vi "Begin.vi"(8 "error in (no error)":errorcluster, 10 "Configuration in":variant, 11 "Power Cell Handler in":refnum<class "Power Cell Handler.lvclass">) -> (0 "error out":errorcluster, 3 "Power Cell Handler out":refnum<class "Power Cell Handler.lvclass">)   [LabVIEW 2019, in "Power Cell Handler.lvlib" / "Power Cell Handler.lvclass"]
uses:
  Power Cell Handler.lvclass
  <vilib>/Rock Robotics/WPI/ThirdParty/Phoenix-LabVIEW/Motor Controller/Controls/CTRE_Phoenix_MotorControl_SupplyCurrentLimitConfiguration.ctl
  Power Cell Handler.lvclass/Power Cell Handler.ctl
  <vilib>/Rock Robotics/WPI/ThirdParty/Phoenix-LabVIEW/Motor Controller/Controls/CTRE_Phoenix_MotorControl_FeedbackDevice_TalonFX.ctl
  <vilib>/Rock Robotics/WPI/ThirdParty/Phoenix-LabVIEW/Motor Controller/Controls/CTRE_Phoenix_MotorControl_TalonFXInvertType.ctl
  <vilib>/Rock Robotics/WPI/ThirdParty/Phoenix-LabVIEW/Motor Controller/Controls/CTRE_Phoenix_MotorControl_FeedbackDevice.ctl
  7b361c19-ac6e-4022-bfe1-45901947c1fc.vi
  19b491db-85f4-4e91-bd7a-c7c0939619b7.vi
  10e73dc3-d3e9-4580-8caf-7344cce1af74.vi
  ea745d27-1b7a-4aa6-8db5-1ac96fa4d0e2.vi
  80b243bf-0e5b-4295-a3d8-317614f9daec.vi
  7ce307d2-5cf6-42cf-8e64-50757e446175.vi
  680ce7d0-c1b2-4c80-9ba9-9f229533ea2f.vi
  848b9887-b104-4cac-9511-37ed5d87697b.vi
  <vilib>/Utility/error.llb/Trim Whitespace.vi
  <vilib>/Utility/error.llb/Error Cluster From Error Code.vi
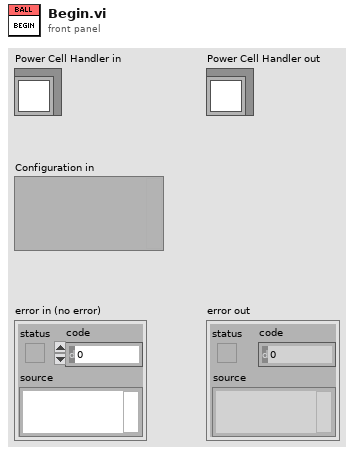
[diagram p1: front panel]
types:
  T1 = typedef "CTRE_Phoenix_MotorControl_SupplyCurrentLimitConfiguration.ctl" = cluster{"Enable?":bool, "Current Limit":dbl, "Threshold Current":dbl, "Threshold Time":dbl}
  T2 = typedef "CTRE_Phoenix_MotorControl_TalonFXInvertType.ctl" = enum16{"Counter-Clockwise", "Clockwise"}
  T3 = typedef "CTRE_Phoenix_MotorControl_FeedbackDevice_TalonFX.ctl" = i8
  T4 = typedef "WPI_MotorControlDeviceRef.ctl" = cluster{"DeviceStatus":errorcluster, "Type":T5, "PWM":cluster{"PWM Channel":T6, "DeadBand":T7}, "CAN":cluster{"Device Number":u8, "SetOutput VI Ref":variant, "GetOutput VI Ref":variant, "Enable VI Ref":variant, "Disable VI Ref":variant, "Data":variant}, "Invert":bool, "DIO PWM":cluster{"PWM \"Enable\" Channel":T6, "DIOChannel":T8, "PWM Rate":dbl}}
  T5 = typedef "WPI_MotorControlType.ctl" = enum16{"PWM", "CAN", "DIO PWM"}
  T6 = typedef "FPGA_DIOPWMChannel.ctl" = enum8{"PWM 0", "PWM 1", "PWM 2", "PWM 3", "PWM 4", "PWM 5", "PWM 6", "PWM 7", "PWM 8", "PWM 9", "PWM MXP 0", "PWM MXP 1", "PWM MXP 2", "PWM MXP 3", "PWM MXP 4", "PWM MXP 5", "PWM MXP 6", "PWM MXP 7", "PWM MXP 8", "PWM MXP 9", "Invalid"}
  T7 = typedef "WPI_PWMDeadband.ctl" = cluster{"Name":string, "maxPositivePwm":i32, "minPositivePwm":i32, "centerPwm":i32, "maxNegativePwm":i32, "minNegativePwm":i32, "angularRange":u16}
  T8 = typedef "FPGA_DIOChannel.ctl" = enum8{"DIO 0", "DIO 1", "DIO 2", "DIO 3", "DIO 4", "DIO 5", "DIO 6", "DIO 7", "DIO 8", "DIO 9", "DIO MXP 0", "DIO MXP 1", "DIO MXP 2", "DIO MXP 3", "DIO MXP 4", "DIO MXP 5", "DIO MXP 6", "DIO MXP 7", "DIO MXP 8", "DIO MXP 9", "DIO MXP 10", "DIO MXP 11", "DIO MXP 12", "DIO MXP 13", "DIO MXP 14", "DIO MXP 15", "SPI Port CS1", "SPI Port CS2", "SPI Port CS3", "SPI Port MISO", "SPI Port MOSI", "Invalid"}
  T9 = typedef "CTRE_Phoenix_MotorControl_FeedbackDevice.ctl" = i8
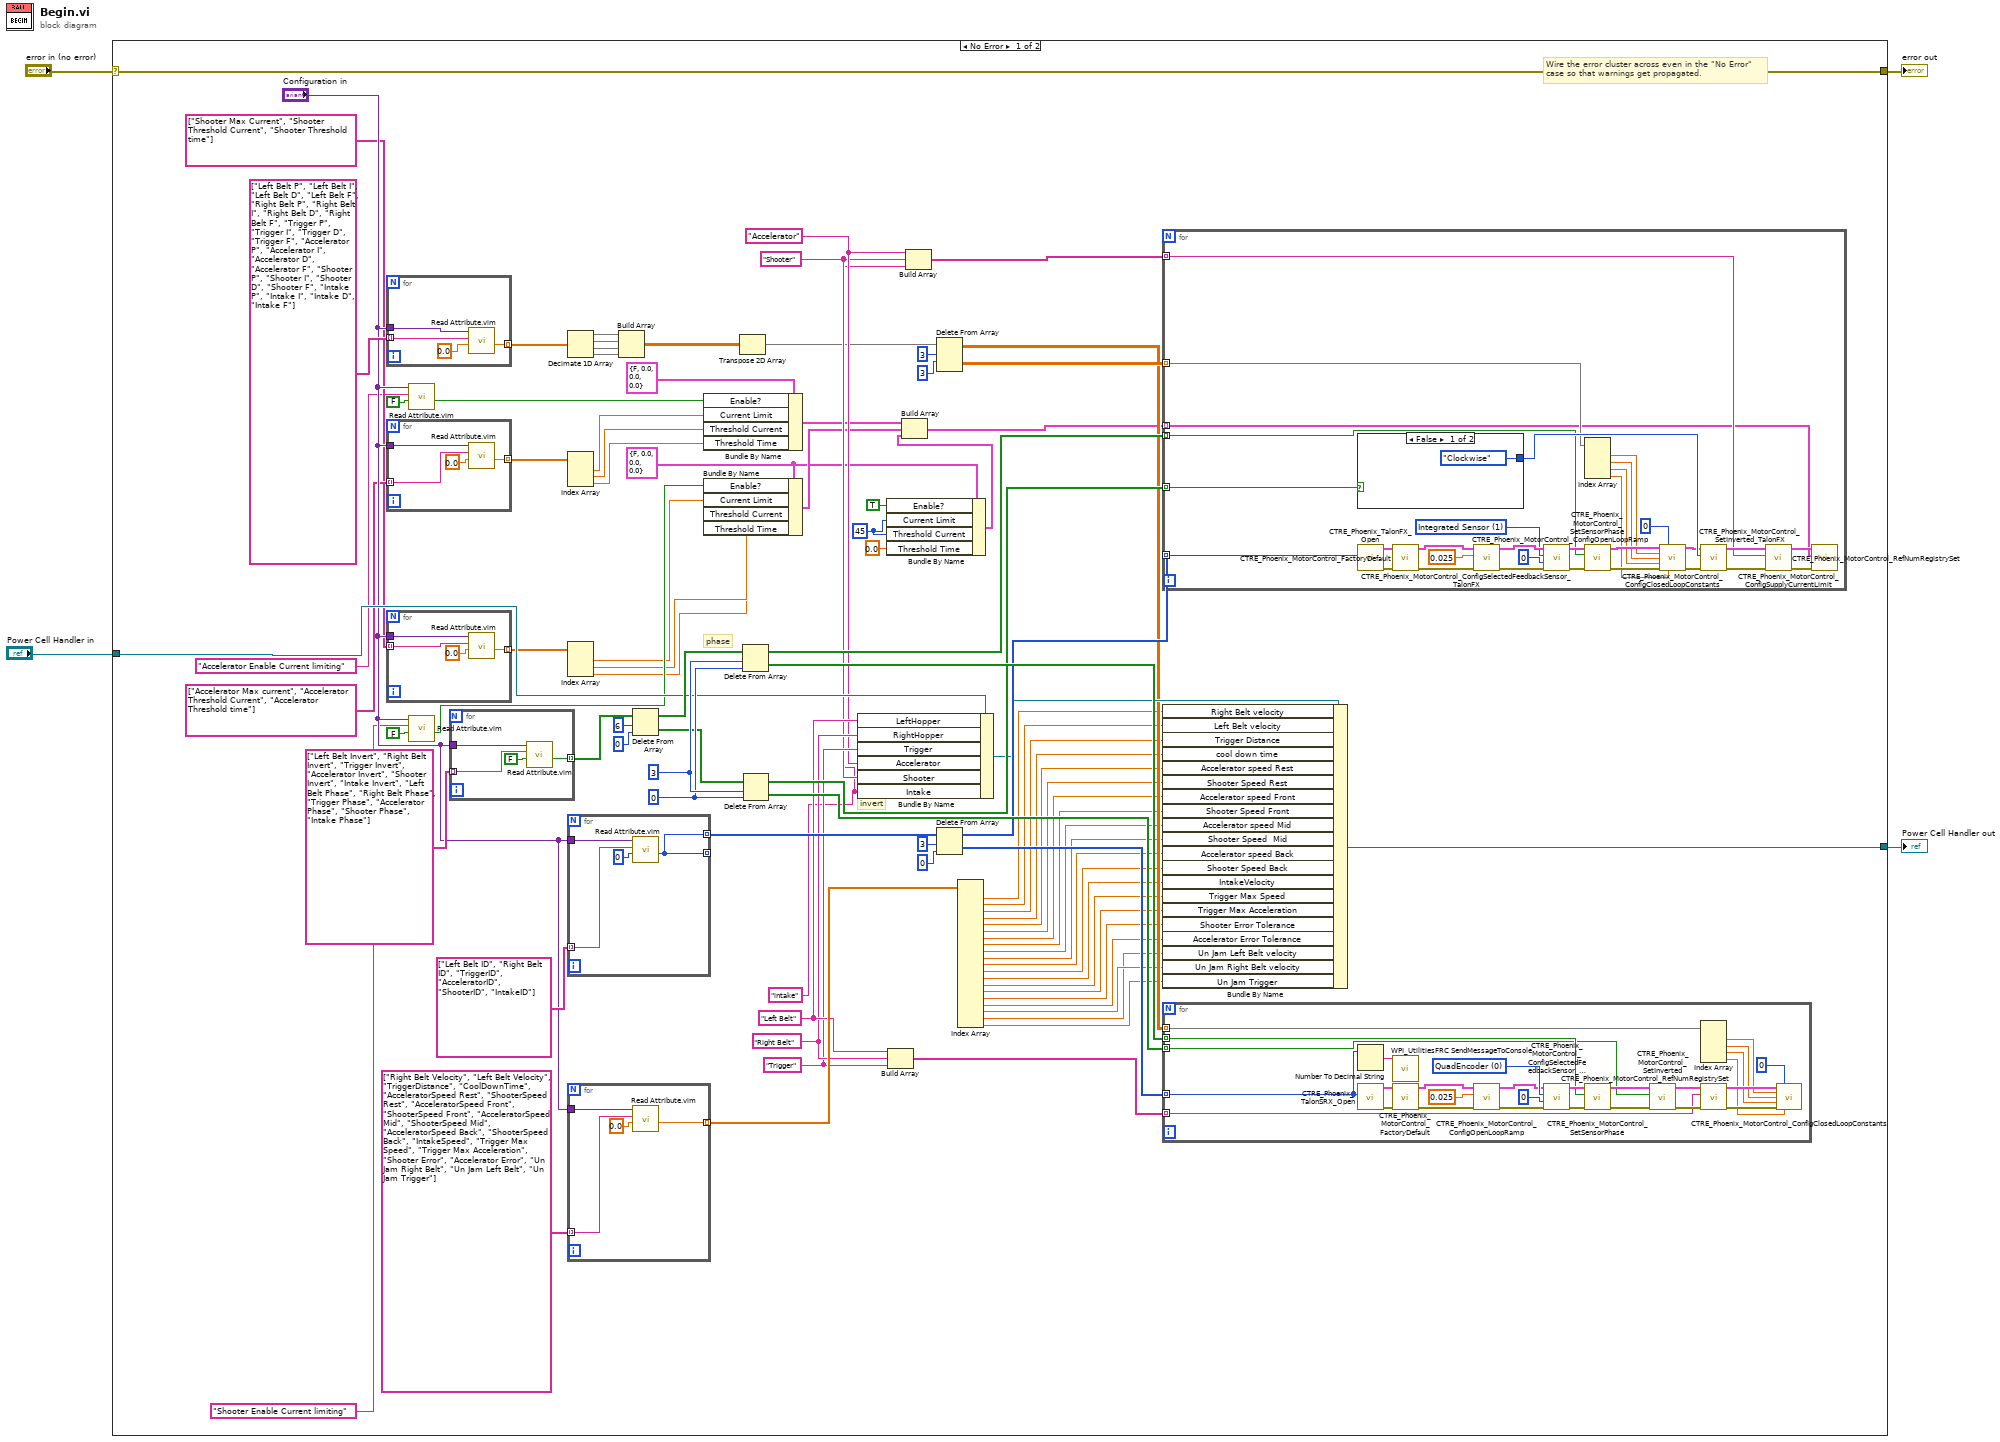
[diagram p0: block diagram]
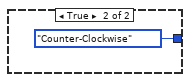
[diagram p2: hidden frame]
diagram:
  n1 = case shown="No Error" "error in (no error)" {
    selector: "error in (no error)" -> [w94 w181]
    tunnel: [w94 w181] -> w3
    tunnel: [w63 w180] -> w1
    tunnel: "Power Cell Handler in" -> [w72 w180]
    frame No Error {
      w8 = 45
      w10 = T1 {"Enable?"=FALSE, "Current Limit"=0.0, "Threshold Current"=0.0, "Threshold Time"=0.0} ("Supply Current Limit Configuration 2")
      w5 = "intake"
      w65 = "Shooter"
      w66 = "Accelerator"
      w68 = "Trigger"
      w69 = "Right Belt"
      w70 = "Left Belt"
      w87 = 3 ("length")
      w86 = 0 ("index")
      # "phase"
      # "invert"
      # "Wire the error cluster across even in the \"No Error\"\ncase so that warnings get propagated."
      n2 = for {
        tunnel: "Configuration in" -> [w118]
        tunnel: string[] ["Left Belt P", "Left Belt I", "Left Belt D", "Left Belt F", "Right Belt P", "Right Belt I", "Right Belt D", "Right Belt F", "Trigger P", "Trigger I", "Trigger D", "Trigger F", "Accelerator P", "Accelerator I", "Accelerator D", "Accelerator F", "Shooter P", "Shooter I", "Shooter D", "Shooter F", "Intake P", "Intake I", "Intake D", "Intake F"] -> [w117] mode=indexing
        tunnel: [w116] -> w62 mode=indexing
        n3 = call "Read Attribute.vim"("default value (data type)"=0.0, "name"=w117, "variant in"=w118) -> ("value"=w116:dbl)  [unwired: 5 in, 3 out]
      }
      n4 = for {
        tunnel: "Configuration in" -> [w102]
        tunnel: [w101] -> w37 mode=indexing
        tunnel: string[] ["Accelerator Max current", "Accelerator Threshold Current", "Accelerator Threshold time"] -> [w99] mode=indexing
        n5 = call "Read Attribute.vim"("default value (data type)"=0.0, "name"=w99, "variant in"=w102) -> ("value"=w101:dbl)  [unwired: 5 in, 3 out]
      }
      n6 = for {
        tunnel: "Configuration in" -> [w98]
        tunnel: [w97] -> w36 mode=indexing
        tunnel: string[] ["Shooter Max Current", "Shooter Threshold Current", "Shooter Threshold time"] -> [w95] mode=indexing
        n7 = call "Read Attribute.vim"("default value (data type)"=0.0, "name"=w95, "variant in"=w98) -> ("value"=w97:dbl)  [unwired: 5 in, 3 out]
      }
      n8 = call "Read Attribute.vim"("default value (data type)"=FALSE, "name"="Accelerator Enable Current limiting", "variant in"="Configuration in") -> ("value"=w30:bool)  [unwired: 5 in, 3 out]
      n9 = call "Read Attribute.vim"("default value (data type)"=FALSE, "name"="Shooter Enable Current limiting", "variant in"="Configuration in") -> ("value"=w29:bool)  [unwired: 5 in, 3 out]
      n10 = for {
        tunnel: "Configuration in" -> [w114]
        tunnel: string[] ["Left Belt Invert", "Right Belt Invert", "Trigger Invert", "Accelerator Invert", "Shooter Invert", "Intake Invert", "Left Belt Phase", "Right Belt Phase", "Trigger Phase", "Accelerator Phase", "Shooter Phase", "Intake Phase"] -> [w113] mode=indexing
        tunnel: [w111] -> w91 mode=indexing
        n11 = call "Read Attribute.vim"("default value (data type)"=FALSE, "name"=w113, "variant in"=w114) -> ("value"=w111:bool)  [unwired: 5 in, 3 out]
      }
      n12 = Decimate 1D Array(w62) -> (w61:dbl[], w60:dbl[], w59:dbl[], w46:dbl[])
      n13 = Index Array(array=w37) -> (element #1=w33:dbl, element #2=w32:dbl, element #3=w31:dbl)  [unwired: 3 in]
      n14 = Index Array(array=w36) -> (element #1=w28:dbl, element #2=w27:dbl, element #3=w26:dbl)  [unwired: 3 in]
      n15 = for {
        tunnel: "Configuration in" -> [w110]
        tunnel: string[] ["Left Belt ID", "Right Belt ID", "TriggerID", "AcceleratorID", "ShooterID", "IntakeID"] -> [w109] mode=indexing
        tunnel: [w108] -> _ mode=indexing
        tunnel: [w108] -> w79 mode=indexing
        n16 = call "Read Attribute.vim"("default value (data type)"=0, "name"=w109, "variant in"=w110) -> ("value"=w108:i32)  [unwired: 5 in, 3 out]
      }
      n17 = for {
        tunnel: "Configuration in" -> [w106]
        tunnel: string[] ["Right Belt Velocity", "Left Belt Velocity", "TriggerDistance", "CoolDownTime", "AcceleratorSpeed Rest", "ShooterSpeed Rest", "AcceleratorSpeed Front", "ShooterSpeed Front", "AcceleratorSpeed Mid", "ShooterSpeed Mid", "AcceleratorSpeed Back", "ShooterSpeed Back", "IntakeSpeed", "Trigger Max Speed", "Trigger Max Acceleration", "Shooter Error", "Accelerator Error", "Un Jam Right Belt", "Un Jam Left Belt", "Un Jam Trigger"] -> [w105] mode=indexing
        tunnel: [w104] -> w73 mode=indexing
        n18 = call "Read Attribute.vim"("default value (data type)"=0.0, "name"=w105, "variant in"=w106) -> ("value"=w104:dbl)  [unwired: 5 in, 3 out]
      }
      n19 = Build Array(w61, w60, w59, w46) -> (w58:dbl[][])
      n20 = Delete From Array(array=w91, length=6, index=0) -> (deleted portion=w85:bool[], array with subset deleted=w88:bool[])
      n21 = Bundle By Name(cluster=T1 {"Enable?"=FALSE, "Current Limit"=0.0, "Threshold Current"=0.0, "Threshold Time"=0.0} ("Supply Current Limit Configuration"), "Enable?"=w30, "Current Limit"=w33, "Threshold Current"=w32, "Threshold Time"=w31) -> (w35:T1)
      n22 = Bundle By Name(cluster=w10, "Enable?"=w29, "Current Limit"=w28, "Threshold Current"=w27, "Threshold Time"=w26) -> (w34:T1)
      n23 = Transpose 2D Array(2D array=w58) -> (transposed array=w53:dbl[][])
      n24 = Delete From Array(array=w88, length=w87, index=w86) -> (deleted portion=w83:bool[], array with subset deleted=w81:bool[])
      n25 = Delete From Array(array=w85, length=w87, index=w86) -> (deleted portion=w84:bool[], array with subset deleted=w82:bool[])
      n26 = Bundle By Name(cluster=w72, "LeftHopper"=w70, "RightHopper"=w69, "Trigger"=w68, "Accelerator"=w66, "Shooter"=w65, "Intake"=w5) -> (w71:refnum<class "Power Cell Handler.lvclass">)
      n27 = Bundle By Name(cluster=w10, "Enable?"=TRUE, "Current Limit"=w8, "Threshold Current"=w8, "Threshold Time"=0.0) -> (w6:T1)
      n28 = Build Array(w70, w69, w68) -> (w67:string[])
      n29 = Build Array(w35, w34, w6) -> (w25:T1[])
      n30 = Build Array(w66, w65, w5) -> (w64:string[])
      n31 = Delete From Array(array=w53, length=3, index (row)=3) -> (deleted portion=w55:dbl[][], array with subset deleted=w54:dbl[][])  [unwired: 1 in]
      n32 = Delete From Array(array=w79, length=3, index=0) -> (deleted portion=w76:i32[], array with subset deleted=w75:i32[])
      n33 = Index Array(array=w73) -> (element #1=w52:dbl, element #2=w51:dbl, element #3=w50:dbl, element #4=w49:dbl, element #5=w48:dbl, element #6=w47:dbl, element #7=w24:dbl, element #8=w23:dbl, element #9=w22:dbl, element #10=w21:dbl, element #11=w20:dbl, element #12=w19:dbl, element #13=w18:dbl, element #14=w17:dbl, element #15=w16:dbl, element #16=w15:dbl, element #17=w14:dbl, element #18=w13:dbl, element #19=w12:dbl, element #20=w11:dbl)  [unwired: 20 in]
      n34 = for {
        tunnel: w55 -> [w127] mode=indexing
        tunnel: w82 -> [w126] mode=indexing
        tunnel: w81 -> [w125] mode=indexing
        tunnel: w75 -> [w124] mode=indexing
        tunnel: w64 -> [w123] mode=indexing
        tunnel: w25 -> [w119] mode=indexing
        w122 = T3 1 items=["Integrated Sensor"=1, "Sensor Sum (S0 + S1)"=9, "Sensor Difference (D0 - D1)"=10, "Remote Source 0"=11, "Remote Source 1"=12, "None"=14, "Software Emulated"=15] ("Talon FX Feedback Device")
        n35 = case shown="False" w126 {
          tunnel: [CTRE_Phoenix_MotorControl_TalonFXInvertType."Clockwise" ("Invert Type") CTRE_Phoenix_MotorControl_TalonFXInvertType."Counter-Clockwise" ("Invert Type")] -> w137
          frame False {
          }
          frame True {
          }
        }
        n36 = call <vilib>:"CTRE_Phoenix_TalonFX_Open.vi"("Device Number"=w124) -> ("error out"=w149:errorcluster, "CAN Talon SRX Ref"=w148:T4)  [unwired: 9 in]
        n37 = call <vilib>:"CTRE_Phoenix_MotorControl_FactoryDefault.vi"("error in"=w149, "PhoenixMotorControlDevRef"=w148) -> ("error out"=w142:errorcluster, "PhoenixMotorControlDevRef"=w143:T4)  [unwired: 8 in]
        n38 = call <vilib>:"CTRE_Phoenix_MotorControl_ConfigOpenLoopRamp.vi"("error in (no error)"=w142, "secondsFromNeutralToFull"=0.025, "PhoenixMotorControlDevRef"=w143) -> ("error out"=w140:errorcluster, "PhoenixMotorControlDevRef"=w141:T4)  [unwired: 7 in]
        n39 = call <vilib>:"CTRE_Phoenix_MotorControl_ConfigSelectedFeedbackSensor_TalonFX.vi"("error in (no error)"=w140, "pidLoopIdx"=0, "Talon FX Feedback Device"=w122, "PhoenixMotorControlDevRef"=w141) -> ("error out"=w145:errorcluster, "PhoenixMotorControlDevRef"=w146:T4)  [unwired: 6 in]
        n40 = Index Array(array=w127) -> (element #1=w131:dbl, element #2=w130:dbl, element #3=w129:dbl, element #4=w128:dbl)  [unwired: 4 in]
        n41 = call <vilib>:"CTRE_Phoenix_MotorControl_SetSensorPhase.vi"("error in (no error)"=w145, "PhaseSensor"=w125, "PhoenixMotorControlDevRef"=w146) -> ("error out"=w135:errorcluster, "PhoenixMotorControlDevRef"=w136:T4)  [unwired: 7 in]
        n42 = call <vilib>:"CTRE_Phoenix_MotorControl_ConfigClosedLoopConstants.vi"("PhoenixMotorControlDevRef"=w136, "slotIdx"=0, "P"=w131, "I"=w130, "D"=w129, "error in (no error)"=w135, "F"=w128) -> ("PhoenixMotorControlDevRef"=w134:T4, "error out"=w133:errorcluster)  [unwired: 7 in]
        n43 = call <vilib>:"CTRE_Phoenix_MotorControl_SetInverted_TalonFX.vi"("error in (no error)"=w133, "Invert Type"=w137, "PhoenixMotorControlDevRef"=w134) -> ("error out"=w139:errorcluster, "PhoenixMotorControlDevRef"=w138:T4)  [unwired: 7 in]
        n44 = call <vilib>:"CTRE_Phoenix_MotorControl_RefNumRegistrySet.vi"("error in (no error)"=w139, "refnum name"=w123, "PhoenixMotorControlDevRef"=w138) -> ("error out"=w120:errorcluster, "PhoenixMotorControlDevRef"=w121:T4)  [unwired: 7 in]
        n45 = call <vilib>:"CTRE_Phoenix_MotorControl_ConfigSupplyCurrentLimit.vi"("error in (no error)"=w120, "Supply Current Limit Configuration"=w119, "PhoenixMotorControlDevRef"=w121) -> ()  [unwired: 7 in, 2 out]
      }
      n46 = Bundle By Name(cluster=w71, "Right Belt velocity"=w52, "Left Belt velocity"=w51, "Trigger Distance"=w50, "cool down time"=w49, "Accelerator speed Rest"=w48, "Shooter Speed Rest"=w47, "Accelerator speed Front"=w24, "Shooter Speed Front"=w23, "Accelerator speed Mid"=w22, "Shooter Speed  Mid"=w21, "Accelerator speed Back"=w20, "Shooter Speed Back"=w19, "IntakeVelocity"=w18, "Trigger Max Speed"=w17, "Trigger Max Acceleration"=w16, "Shooter Error Tolerance"=w15, "Accelerator Error Tolerance"=w14, "Un Jam Left Belt velocity"=w12, "Un Jam Right Belt velocity"=w13, "Un Jam Trigger"=w11) -> (w63:refnum<class "Power Cell Handler.lvclass">)
      n47 = for {
        tunnel: w84 -> [w156] mode=indexing
        tunnel: w83 -> [w157] mode=indexing
        tunnel: w54 -> [w155] mode=indexing
        tunnel: w76 -> [w153] mode=indexing
        tunnel: w67 -> [w154] mode=indexing
        w177 = T9 0 items=["QuadEncoder"=0, "Analog"=2, "Tachometer"=4, "Pulse Width Encoded Position"=8, "Sensor Sum (S0 + S1)"=9, "Sensor Difference (D0 - D1)"=10, "Remote Source 0"=11, "Remote Source 1"=12, "Software Emulated"=15] ("Feedback Device")
        n48 = Number To Decimal String(number=w153) -> (decimal integer string=w152:string)  [unwired: 1 in]
        n49 = call <vilib>:"CTRE_Phoenix_TalonSRX_Open.vi"("Device Number"=w153) -> ("error out"=w176:errorcluster, "CAN Talon SRX Ref"=w175:T4)  [unwired: 9 in]
        n50 = call <vilib>:"WPI_UtilitiesFRC SendMessageToConsole.vi"("Message"=w152) -> ()  [unwired: 14 in, 1 out]
        n51 = call <vilib>:"CTRE_Phoenix_MotorControl_FactoryDefault.vi"("error in"=w176, "PhoenixMotorControlDevRef"=w175) -> ("error out"=w167:errorcluster, "PhoenixMotorControlDevRef"=w168:T4)  [unwired: 8 in]
        n52 = call <vilib>:"CTRE_Phoenix_MotorControl_ConfigOpenLoopRamp.vi"("error in (no error)"=w167, "secondsFromNeutralToFull"=0.025, "PhoenixMotorControlDevRef"=w168) -> ("error out"=w165:errorcluster, "PhoenixMotorControlDevRef"=w166:T4)  [unwired: 7 in]
        n53 = call <vilib>:"CTRE_Phoenix_MotorControl_ConfigSelectedFeedbackSensor_Enhanced.vi"("error in (no error)"=w165, "pidLoopIdx"=0, "Feedback Device"=w177, "PhoenixMotorControlDevRef"=w166) -> ("error out"=w172:errorcluster, "PhoenixMotorControlDevRef"=w173:T4)  [unwired: 6 in]
        n54 = call <vilib>:"CTRE_Phoenix_MotorControl_SetSensorPhase.vi"("error in (no error)"=w172, "PhaseSensor"=w157, "PhoenixMotorControlDevRef"=w173) -> ("error out"=w170:errorcluster, "PhoenixMotorControlDevRef"=w171:T4)  [unwired: 7 in]
        n55 = call <vilib>:"CTRE_Phoenix_MotorControl_SetInverted.vi"("error in (no error)"=w170, "Invert?"=w156, "PhoenixMotorControlDevRef"=w171) -> ("error out"=w178:errorcluster, "PhoenixMotorControlDevRef"=w179:T4)  [unwired: 7 in]
        n56 = Index Array(array=w155) -> (element #1=w162:dbl, element #2=w161:dbl, element #3=w160:dbl, element #4=w159:dbl)  [unwired: 4 in]
        n57 = call <vilib>:"CTRE_Phoenix_MotorControl_RefNumRegistrySet.vi"("error in (no error)"=w178, "refnum name"=w154, "PhoenixMotorControlDevRef"=w179) -> ("error out"=w163:errorcluster, "PhoenixMotorControlDevRef"=w164:T4)  [unwired: 7 in]
        n58 = call <vilib>:"CTRE_Phoenix_MotorControl_ConfigClosedLoopConstants.vi"("PhoenixMotorControlDevRef"=w164, "slotIdx"=0, "P"=w162, "I"=w161, "D"=w160, "error in (no error)"=w163, "F"=w159) -> ()  [unwired: 7 in, 2 out]
      }
    }
    frame Error {
    }
  }
  "error out" <- w3
  "Power Cell Handler out" <- w1
